vi "无协议模式（广播）.vi"(8 "错误输入（无错误）":errorcluster, 10 "等待时间（毫秒）":u32, 11 "VISA资源名称":refnum<visa-resource-name>) -> (0 "错误输出":errorcluster, 1 "通讯数据":string, 3 "VISA资源名称输出":refnum<visa-resource-name>)   [LabVIEW 2017]
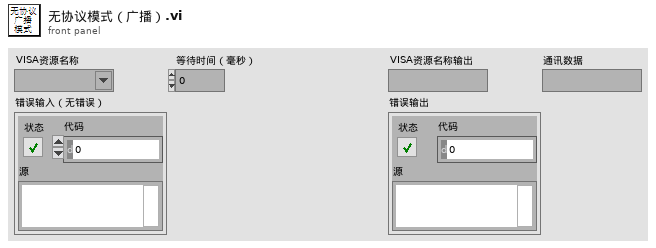
[diagram p1: front panel]
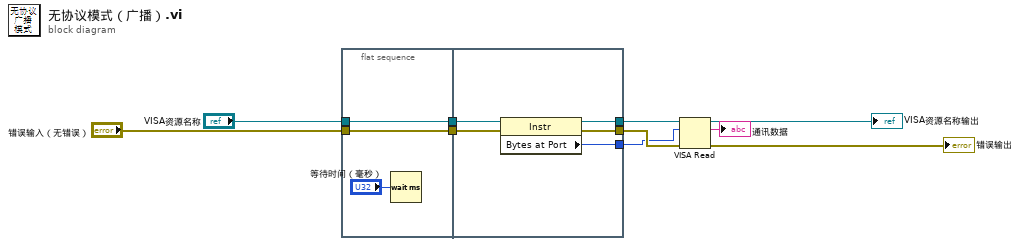
[diagram p0: block diagram]
diagram:
  n1 = flat-sequence {
    tunnel: [w12] -> w10
    tunnel: "VISA资源名称" -> [w12]
    tunnel: "错误输入（无错误）" -> [w11]
    tunnel: [w11] -> w7
    tunnel: w10 -> [w18]
    tunnel: w7 -> [w17]
    tunnel: [w16] -> w6
    tunnel: [w15] -> w5
    tunnel: [w14] -> w4
    frame #0 {
      n2 = Wait (ms)(milliseconds to wait="等待时间（毫秒）") -> ()  [unwired: 1 out]
    }
    frame #1 {
      n3 = property class="Instr"(reference=w18, error in=w17) -> (reference out=w16:refnum<visa-resource-name>, error out=w15:errorcluster, "Bytes at Port"=w14:u32)
    }
  }
  n4 = VISA Read(VISA resource name=w6, byte count=w4, error in (no error)=w5) -> (VISA resource name out=→"VISA资源名称输出":refnum<visa-resource-name>, read buffer=→"通讯数据":string, error out=→"错误输出":errorcluster)  [unwired: 1 out]
